vi "AdventofCodeDay1.vi"() -> ()   [LabVIEW 2019]
panel:
  out "Solution 2":dbl
  out "Solution 1":dbl
  in  "String":string
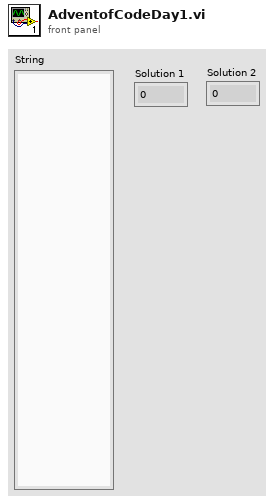
[diagram p1: front panel]
types:
  T1 = enum16{"Native", "Native Command Line", "UNIX", "Macintosh", "DOS"}
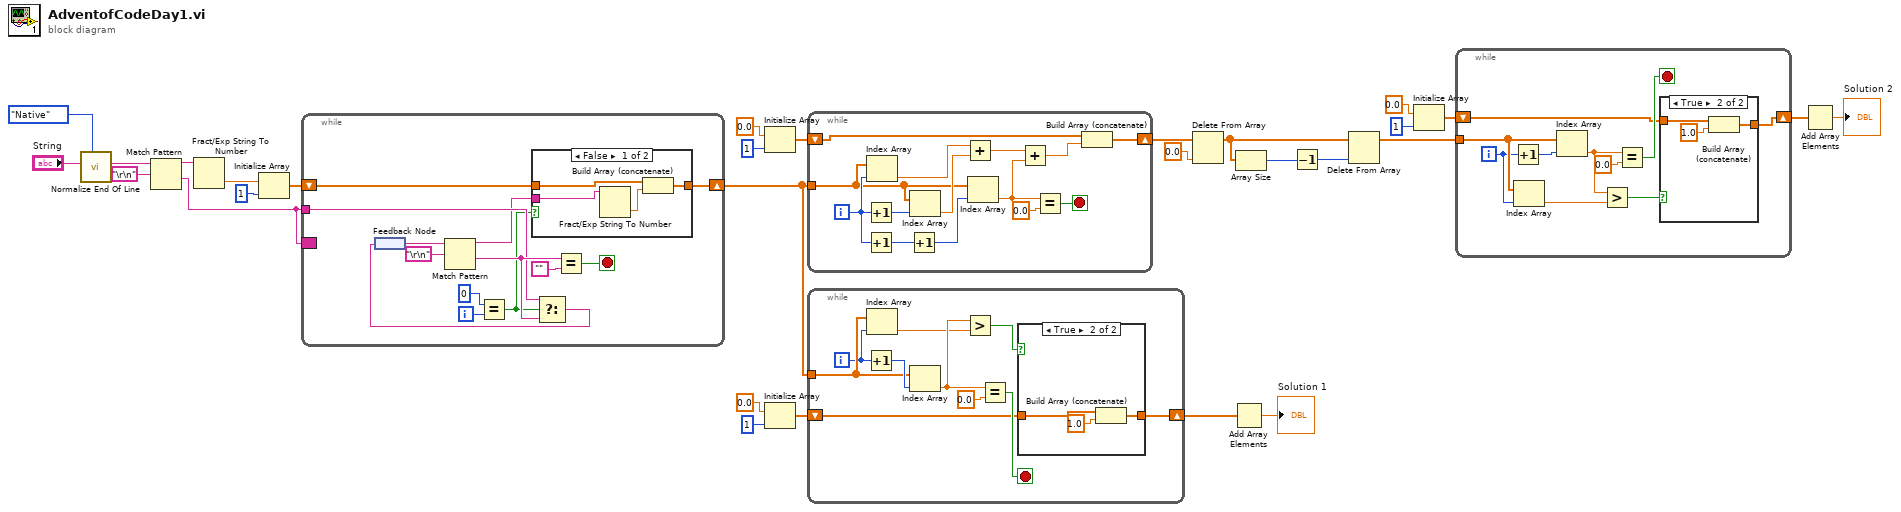
[diagram p0: block diagram]
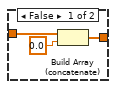
[diagram p2: hidden frame]
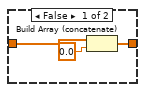
[diagram p3: hidden frame]
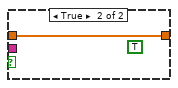
[diagram p4: hidden frame]
diagram:
  n1 = call <vilib>:"Normalize End Of Line.vi"("end of line (Native)"=T1."Native", "string in"="String") -> ("string out"=w28:string)  [unwired: 6 in]
  n2 = Match Pattern(string=w28, regular expression="\r\n") -> (before substring=w23:string, after substring=w21:string)  [unwired: 1 in, 2 out]
  n3 = Fract/Exp String To Number(string=w23) -> (number=w25:dbl)  [unwired: 3 in, 1 out]
  n4 = Initialize Array(w25, 1 ("dimension size")) -> (w22:dbl[])
  n5 = while {
    shift-right: [w30] -> w15
    shift-left: w22 -> [w31]
    tunnel: w21 -> [w38]
    border: w21 -> [_]
    i -> [w35]
    stop <- w40 stop-if-true
    n6 = feedback #1() -> (w36:string)
    n7 = Match Pattern(string=w36, regular expression="\r\n") -> (before substring=w33:string, after substring=w39:string)  [unwired: 1 in, 2 out]
    n8 = Equal?(x=0 ("y"), y=w35) -> (x = y?=w32:bool)
    n9 = case shown="False" w32 {
      tunnel: w33 -> [w46 _]
      tunnel: w31 -> [w45 w47]
      tunnel: [w43 w47] -> w30
      frame False {
        n10 = Fract/Exp String To Number(string=w46) -> (number=w44:dbl)  [unwired: 3 in, 1 out]
        n11 = Build Array (concatenate)(w45, w44) -> (w43:dbl[])
      }
      frame True {
        (unwired) TRUE ("use system decimal point (T)")
      }
    }
    n12 = Select(t=w38, s=w32, f=w39) -> (s? t:f=w37:string)
    n13 = feedback-in #1(w37) -> ()
    n14 = Equal?(x=w39, y="") -> (x = y?=w40:bool)
  }
  n15 = Initialize Array(0.0 ("element"), 1 ("dimension size")) -> (w12:dbl[])
  n16 = Initialize Array(0.0 ("element"), 1 ("dimension size")) -> (w20:dbl[])
  n17 = while {
    tunnel: w15 -> [w54]
    shift-right: [w48] -> w11
    shift-left: w12 -> [w50]
    i -> [w58]
    stop <- w51 stop-if-true
    n18 = Increment(x=w58) -> (x+1=w59:i32)
    n19 = Increment(x=w58) -> (x+1=w60:i32)
    n20 = Index Array(array=w54, index=w58) -> (element=w57:dbl)
    n21 = Increment(x=w60) -> (x+1=w61:i32)
    n22 = Index Array(array=w54, index=w59) -> (element=w56:dbl)
    n23 = Add(x=w57, y=w56) -> (x+y=w55:dbl)
    n24 = Index Array(array=w54, index=w61) -> (element=w52:dbl)
    n25 = Add(x=w55, y=w52) -> (x+y=w49:dbl)
    n26 = Equal?(x=w52, y=0.0) -> (x = y?=w51:bool)
    n27 = Build Array (concatenate)(w50, w49) -> (w48:dbl[])
  }
  n28 = while {
    tunnel: w15 -> [w65]
    shift-right: [w63] -> w17
    shift-left: w20 -> [w62]
    i -> [w64]
    stop <- w70 stop-if-true
    n29 = Increment(x=w64) -> (x+1=w69:i32)
    n30 = Index Array(array=w65, index=w64) -> (element=w67:dbl)
    n31 = Index Array(array=w65, index=w69) -> (element=w68:dbl)
    n32 = Greater?(x=w68, y=w67) -> (0:w66:bool)
    n33 = Equal?(x=w68, y=0.0) -> (x = y?=w70:bool)
    n34 = case shown="True" w66 {
      tunnel: [w72 w75] -> w63
      tunnel: w62 -> [w73 w76]
      frame False {
        n35 = Build Array (concatenate)(w73, 0.0) -> (w72:dbl[])
      }
      frame True {
        n36 = Build Array (concatenate)(w76, 1.0) -> (w75:dbl[])
      }
    }
  }
  n37 = Delete From Array(array=w11, index=0.0) -> (array with subset deleted=w3:dbl[])  [unwired: 1 in, 1 out]
  n38 = Add Array Elements(numeric array=w17) -> (sum=→"Solution 1":dbl)
  n39 = Array Size(array=w3) -> (size(s)=w2:i32)
  n40 = Decrement(x=w2) -> (x-1=w1:i32)
  n41 = Delete From Array(array=w3, index=w1) -> (array with subset deleted=w4:dbl[])  [unwired: 1 in, 1 out]
  n42 = Initialize Array(0.0 ("element"), 1 ("dimension size")) -> (w9:dbl[])
  n43 = while {
    tunnel: w4 -> [w81]
    shift-right: [w79] -> w6
    shift-left: w9 -> [w78]
    i -> [w80]
    stop <- w86 stop-if-true
    n44 = Increment(x=w80) -> (x+1=w85:i32)
    n45 = Index Array(array=w81, index=w80) -> (element=w83:dbl)
    n46 = Index Array(array=w81, index=w85) -> (element=w84:dbl)
    n47 = Greater?(x=w84, y=w83) -> (0:w82:bool)
    n48 = Equal?(x=w84, y=0.0) -> (x = y?=w86:bool)
    n49 = case shown="True" w82 {
      tunnel: [w88 w91] -> w79
      tunnel: w78 -> [w89 w92]
      frame False {
        n50 = Build Array (concatenate)(w89, 0.0) -> (w88:dbl[])
      }
      frame True {
        n51 = Build Array (concatenate)(w92, 1.0) -> (w91:dbl[])
      }
    }
  }
  n52 = Add Array Elements(numeric array=w6) -> (sum=→"Solution 2":dbl)
